vi "F Dwf Analog In Buffer Size Info.vi"(8 "error in (no error)":errorcluster, 9 "pnSizeMax":i32, 10 "pnSizeMin":i32, 11 "hdwf":i32) -> (0 "error out":errorcluster, 1 "pnSizeMax out":i32, 2 "pnSizeMin out":i32, 3 "function return":i32)   [LabVIEW 2021, in "Olasdwf.lvlib"]
doc: "DWFAPI int FDwfAnalogInBufferSizeInfo(HDWF hdwf, int *pnSizeMin, int *pnSizeMax);"
uses:
  Olasdwf.lvlib
  Windows/System32/dwf.dll
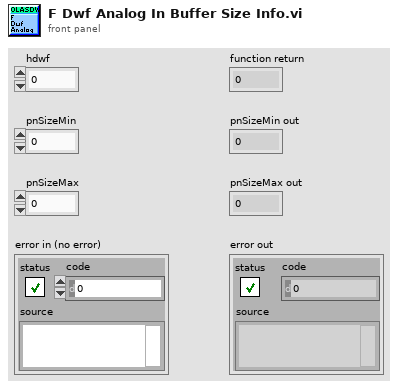
[diagram p1: front panel]
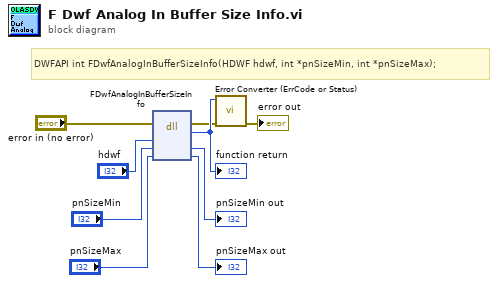
[diagram p0: block diagram]
diagram:
  # "DWFAPI int FDwfAnalogInBufferSizeInfo(HDWF hdwf, int *pnSizeMin, int *pnSizeMax);"
  n1 = dll-call lib="/Windows/System32/dwf.*" fn="FDwfAnalogInBufferSizeInfo"(error in="error in (no error)", "hdwf"="hdwf", "pnSizeMin"="pnSizeMin", "pnSizeMax"="pnSizeMax") -> (error out=w2:errorcluster, w9:i32, "pnSizeMin"=→"pnSizeMin out":i32, "pnSizeMax"=→"pnSizeMax out":i32)  [unwired: 3 in, 1 out]
  "function return" <- w9
  n2 = call "Error Converter (ErrCode or Status).vi"("error in (no error)"=w2, "error code"=w9) -> ("error out"=→"error out":errorcluster)  [unwired: 9 in]
